vi "SPI_Regs.vi"() -> (0 "Init Data Out":u8[](array[numeric]))   [LabVIEW 2018]
panel:
  in  "Регистры":u8[](array[numeric])=[119, 12, 0, 1, 0, 0, 1, 0, 0, 0, 0, 0, 171, 23, 1, 0, 0, 4, 0, 24, 0, 120, 15, 0, 0, 0, 0, 0, 0, 0, 0, 0, 0, 0, 0, 0, 0, 0, 0, 0, 0, 0, 0, 0, 0, 0, 0, 0, 0, 0, 0, 0, 0, 0, 0, 0, 0, 0, 0, 0, 0, 0, 0, 0, 0, 0, 0, 0, 0, 0, 0, 0, 0, 0, 0, 0, 0, 0, 0, 0, 0, 0, 0, 172, 23, 0, 0, 6, 4, 4, 4, 196, 0, 32, 32, 4, 0, 5, 0, 5, 1, 4, 0, 139, 21, 255, 7, 1, 0, 0, 134, 1, 144, 2, 12, 0, 1, 236, 245, 255, 255, 114, 252, 255, 255, 255, 255, 255, 255, 255, 255, 255, 255, 255, 255, 255, 255, 255, 255, 255, 255, 118, 253, 255, 255, 255, 255, 255, 255, 255, 255, 249, 52, 244, 255, 255, 255, 255, 255, 255, 255, 255, 255, 255, 255, 255, 169, 252, 159, 202, 255, 217, 252, 159, 205, 255, 118, 253, 255, 255, 255, 118, 253, 255, 255, 255, 118, 253, 255, 255, 255, 118, 253, 255, 255, 255, 5, 196, 179, 79, 92, 5, 196, 179, 79, 92, 1, 12, 176, 192, 19, 105, 204, 245, 192, 20, 123, 220, 245, 196, 20, 115, 229, 213, 197, 255, 91, 124, 49, 192, 2, 87, 140, 241, 192, 19, 123, 220, 85, 68, 47, 5, 0, 241, 255, 255, 255, 255, 95, 192, 14, 5, 236, 0, 0, 0, 0, 0, 0, 0, 0, 0, 0, 0, 0, 0, 0, 0, 0, 0, 0, 0, 0, 0, 0, 0, 0, 0, 0, 0, 0, 0, 0, 0, 0, 0, 0, 0, 0, 0, 0, 0, 0, 0, 0, 0, 0, 0, 0, 0, 0, 0, 0, 0, 0, 0, 0, 0, 106, 1, 0, 0, 6, 27, 142, 9, 108, 57, 0, 0, 0, 0, 108, 57, 23, 15, 8, 1, 20, 0, 56, 71, 96, 68, 0, 0, 0, 0, 188, 194, 172, 160, 180, 148, 148, 200, 0, 160, 128, 148, 194, 66, 66, 64, 0, 0, 254, 254, 254, 254, 254, 254, 16, 160, 192, 0, 0, 0, 0, 0]
  # "For Initialization VI requirements and help, please read directions located on Block Diagram."
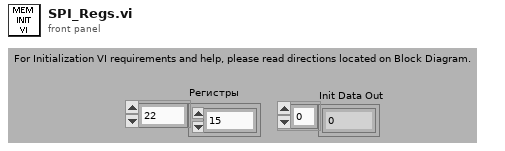
[diagram p1: front panel]
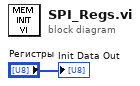
[diagram p0: block diagram]
diagram:
  "Init Data Out" <- "Регистры"
